vi "CenterOfGravityCalc.vi"(7 "clustPointagFin":T1, 11 "error in (no error)":errorcluster) -> (8 "clustPointagFin":T1, 15 "error out":errorcluster)   [LabVIEW 2020, in "Acquisition.lvlib"]
doc: "Perform the acquisition. Replace the contents of this diagram with calls to acquisition hardware."
uses:
  Acquisition.lvlib
  SETTING/clustOA.ctl
  <vilib>/Analysis/Matrix/Datatypes/RealMatrix.ctl
  <vilib>/Analysis/Matrix/NI_Matrix.lvlib
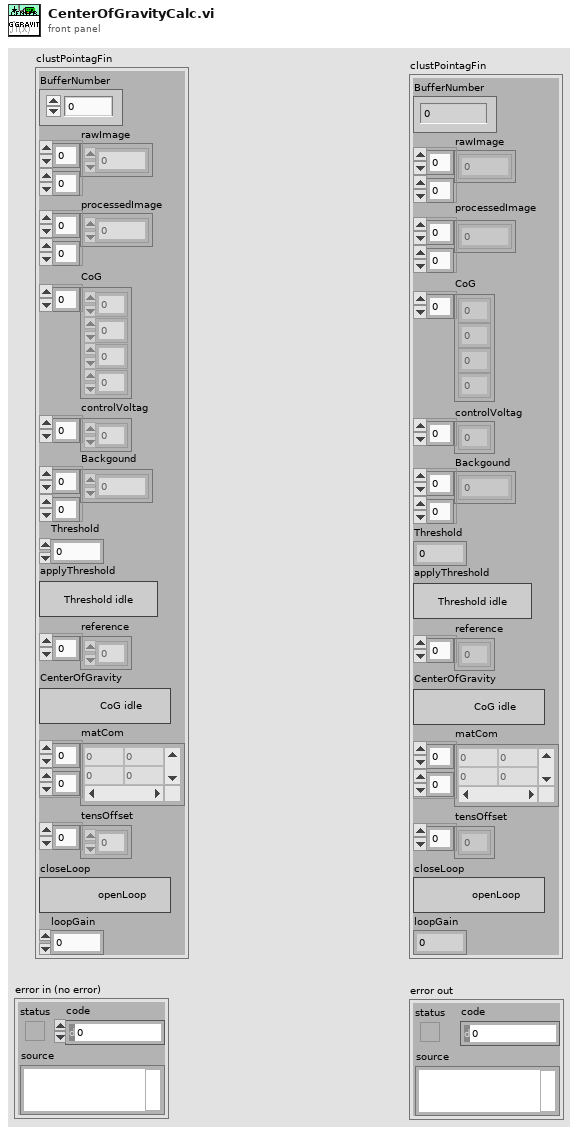
[diagram p1: front panel]
types:
  T1 = typedef "clustOA.ctl" = cluster{"BufferNumber":u32, "rawImage":u16[][], "processedImage":sgl[][], "CoG":dbl[], "controlVoltag":dbl[], "Backgound":sgl[][], "Threshold":dbl, "applyThreshold":bool, "reference":dbl[], "CenterOfGravity":bool, "matCom":T2, "tensOffset":dbl[], "closeLoop":bool, "loopGain":dbl}
  T2 = typedef "NI_Matrix.lvlib/RealMatrix.ctl" = dbl[][]
  T3 = enum16{"Initialisation", "Calcul CdG a", "Calcul CdG b"}
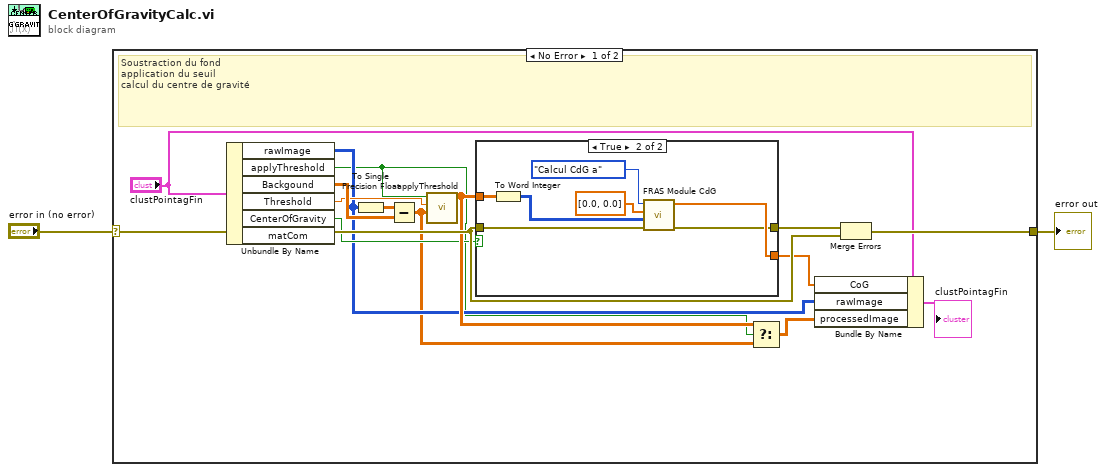
[diagram p0: block diagram]
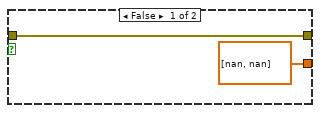
[diagram p2: hidden frame]
diagram:
  n1 = case shown="No Error" "error in (no error)" {
    selector: "error in (no error)" -> [w11 w27]
    tunnel: [w17 w27] -> w1
    frame No Error {
      # "Soustraction du fond\napplication du seuil\ncalcul du centre de gravité"
      n2 = Unbundle By Name("clustPointagFin") -> ("rawImage"=w5:u16[][], "applyThreshold"=w3:bool, "Backgound"=w15:sgl[][], "Threshold"=w14:dbl, "CenterOfGravity"=w6:bool)  [unwired: 1 out]
      n3 = To Single Precision Float(number=w5) -> (single precision float=w16:sgl[][])
      n4 = Subtract(x=w16, y=w15) -> (x-y=w4:sgl[][])
      n5 = call "applyThreshold.vi"("inIma"=w4, "valSeuil"=w14, "applyThreshold"=w3) -> ("imaOut"=w7:sgl[][])  [unwired: 8 in]
      n6 = case shown="True" w6 {
        tunnel: w11 -> [w18 w26]
        tunnel: [dbl[] [nan, nan] ("array") w25] -> w9
        tunnel: w7 -> [_ w20]
        tunnel: [w18 w21] -> w10
        frame False {
        }
        frame True {
          n7 = To Word Integer(number=w20) -> (16bit integer=w23:i16[][])
          n8 = call "FRAS Module CdG.vi"("error in"=w26, "Imagette seuillée"=w23, "inCdG[Pixels]"=dbl[] [0.0, 0.0], "Mode CdG"=T3."Calcul CdG a") -> ("error out"=w21:errorcluster, "CdGOut [Pixels]"=w25:dbl[])  [unwired: 5 in]
        }
      }
      n9 = Select(t=w7, s=w3, f=w4) -> (s? t:f=w8:sgl[][])
      n10 = Bundle By Name(cluster="clustPointagFin", "CoG"=w9, "rawImage"=w5, "processedImage"=w8) -> (→"clustPointagFin":T1)
      n11 = Merge Errors(w10, w11) -> (w17:errorcluster)
    }
    frame Error {
    }
  }
  "error out" <- w1
